vi "Communication - Zero Data (FGV).vi"(7 "Action":T1=enum."Write", 8 "error in (no error)":errorcluster, 11 "Zero":dbl[](array[numeric])) -> (0 "error out":errorcluster, 3 "Zero Out":dbl[](array[numeric]))   [LabVIEW 2019]
uses:
  Controls/FGV States.ctl
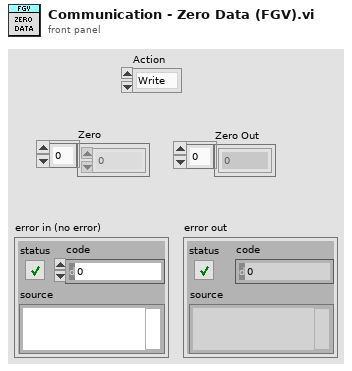
[diagram p1: front panel]
types:
  T1 = typedef "FGV States.ctl" = enum16{"Read", "Write"}
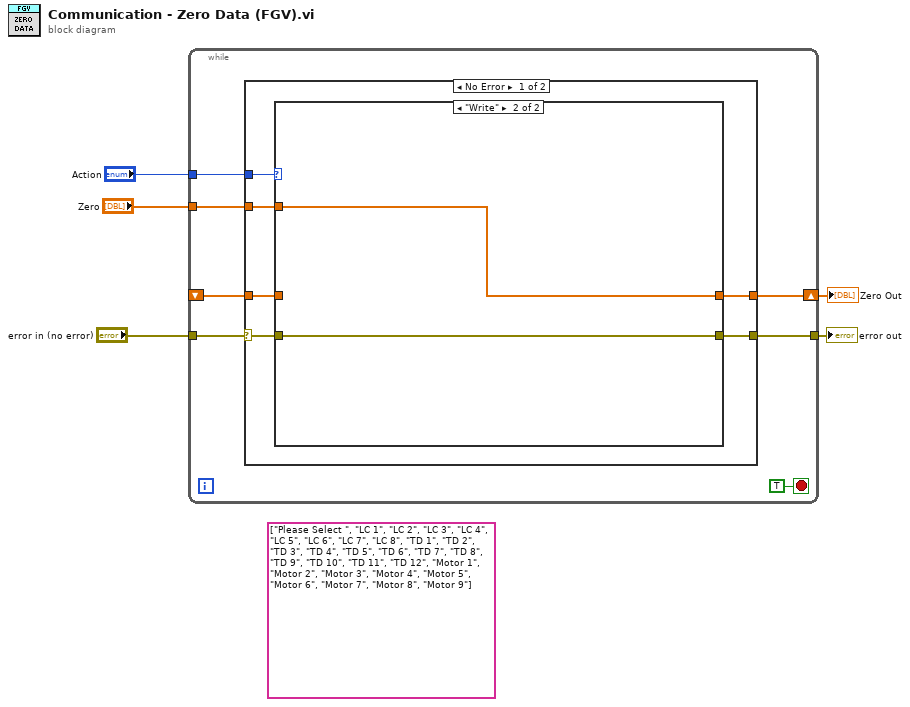
[diagram p0: block diagram]
diagram:
  (unwired) string[] ["Please Select ", "LC 1", "LC 2", "LC 3", "LC 4", "LC 5", "LC 6", "LC 7", "LC 8", "TD 1", "TD 2", "TD 3", "TD 4", "TD 5", "TD 6", "TD 7", "TD 8", "TD 9", "TD 10", "TD 11", "TD 12", "Motor 1", "Motor 2", "Motor 3", "Motor 4", "Motor 5", "Motor 6", "Motor 7", "Motor 8", "Motor 9"] ("string")
  n1 = while {
    tunnel: "Action" -> [w12]
    tunnel: "Zero" -> [w10]
    shift-right: [w11] -> w3
    shift-left: _ -> [w9]
    tunnel: "error in (no error)" -> [w7]
    tunnel: [w6] -> w1
    stop <- TRUE stop-if-true
    n2 = case shown="No Error" w7 {
      selector: w7 -> [w13 w23]
      tunnel: w12 -> [w18 _]
      tunnel: [w17 w24] -> w11
      tunnel: w10 -> [w16 _]
      tunnel: w9 -> [w15 w24]
      tunnel: [w14 w23] -> w6
      frame No Error {
        n3 = case shown="\"Write\"" w18 {
          tunnel: [w20 w22] -> w17
          tunnel: w16 -> [_ w22]
          tunnel: w15 -> [w20 _]
          tunnel: [w19 w21] -> w14
          tunnel: w13 -> [w19 w21]
          frame "Read", Default {
          }
          frame "Write" {
          }
        }
      }
      frame Error {
      }
    }
  }
  "Zero Out" <- w3
  "error out" <- w1
